vi "ReadAnalogChannel.vi"(8 "error in (no error)":errorcluster, 11 "Oscilloscope in":refnum<class "Oscilloscope.lvclass">) -> (0 "error out":errorcluster, 3 "Oscilloscope out":refnum<class "Oscilloscope.lvclass">)   [LabVIEW 2020, in "Oscilloscope.lvclass"]
uses:
  Oscilloscope.lvclass
  C:/Code Projects/CircuitExplorer/AnalogDiscoveryFunction/AnalogDiscoveryFunction.lvclass
  AnalogDiscoveryFunction/AnalogDiscoveryFunction.lvclass/AnalogDiscoveryFunction.ctl
  Oscilloscope.lvclass/Oscilloscope.ctl
  AnalogDiscoveryFunction/GetInstrumentHandle.vi
  <vilib>/DigilentWF/DigilentWF.lvlib
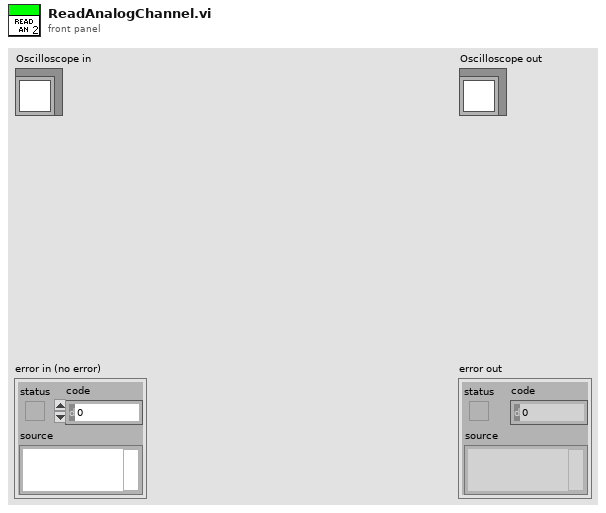
[diagram p1: front panel]
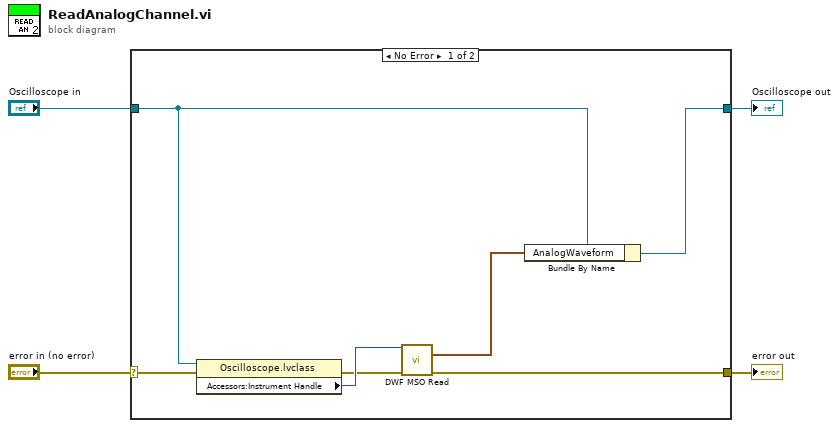
[diagram p0: block diagram]
diagram:
  n1 = case shown="No Error" "error in (no error)" {
    selector: "error in (no error)" -> [w11 w13]
    tunnel: [w6 w13] -> w3
    tunnel: [w5 w12] -> w1
    tunnel: "Oscilloscope in" -> [w8 w12]
    frame No Error {
      n2 = property class="Oscilloscope.lvclass"(reference=w8, error in=w11) -> (error out=w9:errorcluster, "Accessors:Instrument Handle"=w10:u32)  [unwired: 1 out]
      n3 = call <vilib>:"DWF MSO Read.vi"("Instrument Handle In"=w10, "Error In"=w9) -> ("Analog Waveforms"=w7:waveform(dbl)[], "Error Out"=w6:errorcluster)  [unwired: 8 in, 4 out]
      n4 = Bundle By Name(cluster=w8, "AnalogWaveform"=w7) -> (w5:refnum<class "Oscilloscope.lvclass">)
    }
    frame Error {
    }
  }
  "error out" <- w3
  "Oscilloscope out" <- w1
